vi "CSMOMgr-Get CSMO.vi"(6 "GenError? (T)":bool=TRUE, 8 "Error In":errorcluster caption="error in (no error)", 10 "Queue Name":string, 11 "CSMOMgr":T6) -> (0 "error out":errorcluster, 1 "Values":T1={"info"={"Module Name"="", "Requested Name"="", "Group Name"="", "Mode"=enum."Stand Alone", "Allowed Messages"=[]}, "Refs"={"WatchDogQ"=refnum, "CSMDataDVR"=refnum, "Queue"={"HPriorityQ"=refnum, "LowPriorityQ"=refnum}, "GroupDataDVR"=refnum, "TagMap"=refnum, "ExitEvent"=refnum, "NewStateEvent"=refnum, "StatusEvent"=refnum, "InterruptEvent"=refnum}}, 2 "Found":bool, 3 "CSMOMgr Out":T6)   [LabVIEW 2017, in "Communicable State Machine.lvlib"]
uses:
  Communicable State Machine.lvlib
  Def-CSMOMgr.ctl
  CSMQ/_CSMObj.ctl
  CSMQ/_CSMObj-Info.ctl
  Typedef/_CSM_MODE.ctl
  CSMQ/_CSMObj-Refs.ctl
  CSMQ/_CSMObj-Data.ctl
  Priority Queue/Priority Queue.ctl
  Typedef/_Cross CSM State Data.ctl
  Typedef/_CSM_MSG_TYPE.ctl
  Typedef/_Cross CSM State Response.ctl
  Typedef/_CSM_Response Source Message.ctl
  Priority Queue/def-Data(LowPRI-Q).ctl
  CSMQ/_CSMObj-ModeData.ctl
  Typedef/_CSM Status Change Event Data.ctl
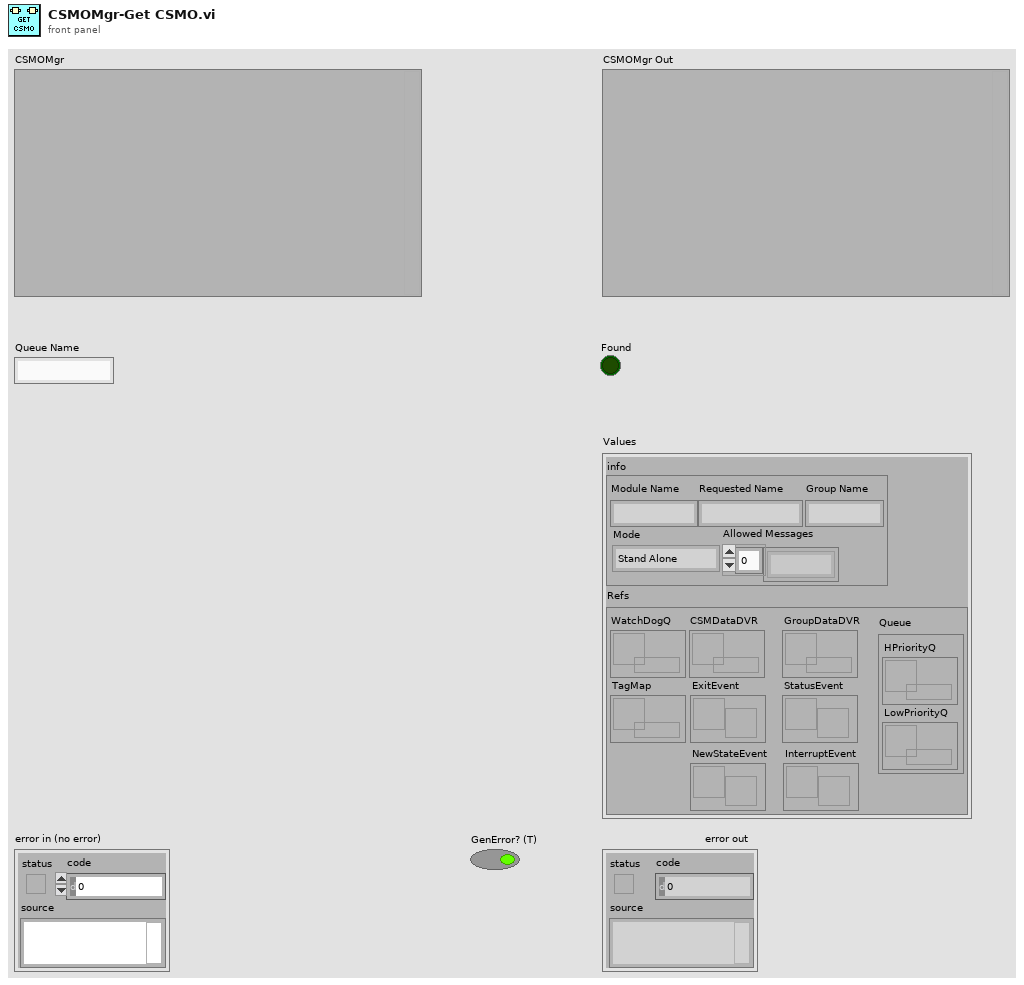
[diagram p1: front panel]
types:
  T1 = typedef "Communicable State Machine.lvlib/_CSMObj.ctl" = cluster{"info":T2, "Refs":T4}
  T2 = typedef "Communicable State Machine.lvlib/_CSMObj-Info.ctl" = cluster{"Module Name":string, "Requested Name":string, "Group Name":string, "Mode":T3, "Allowed Messages":string[]}
  T3 = typedef "Communicable State Machine.lvlib/_CSM_MODE.ctl" = enum16{"Not Exist", "Stand Alone", "CSM", "Worker", "Worker Agent", "Chain Node", "Chain"}
  T4 = typedef "Communicable State Machine.lvlib/_CSMObj-Refs.ctl" = cluster{"WatchDogQ":refnum<queue>, "CSMDataDVR":refnum<data-value>, "Queue":T5, "GroupDataDVR":refnum<data-value>, "TagMap":refnum<data-value>, "ExitEvent":refnum<user-event>, "NewStateEvent":refnum<user-event>, "StatusEvent":refnum<user-event>, "InterruptEvent":refnum<user-event>}
  T5 = typedef "Communicable State Machine.lvlib/Priority Queue.ctl" = cluster{"HPriorityQ":refnum<queue>, "LowPriorityQ":refnum<queue>}
  T6 = typedef "Communicable State Machine.lvlib/Def-CSMOMgr.ctl" = variant
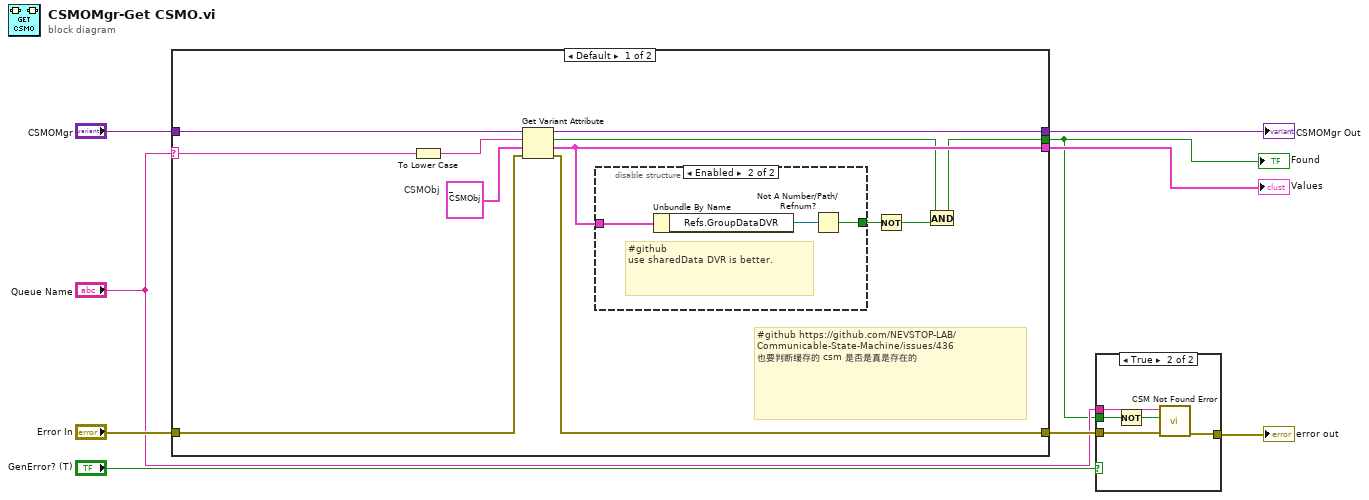
[diagram p0: block diagram]
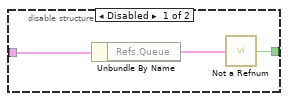
[diagram p3: hidden frame]
diagram:
  n1 = case shown="Default" "Queue Name" {
    selector: "Queue Name" -> [w16 _]
    tunnel: "CSMOMgr" -> [w21 w29]
    tunnel: [w20 w29] -> w8
    tunnel: "Error In" -> [w19 w28]
    tunnel: [w17 w28] -> w6
    tunnel: [w14 _] -> w4
    tunnel: [w13 _] -> w2
    frame Default {
      w18 = T1 {"info"={"Module Name"="", "Requested Name"="", "Group Name"="", "Mode"=enum."Not Exist", "Allowed Messages"=[]}, "Refs"={"WatchDogQ"=refnum, "CSMDataDVR"=refnum, "Queue"={"HPriorityQ"=refnum, "LowPriorityQ"=refnum}, "GroupDataDVR"=refnum, "TagMap"=refnum, "ExitEvent"=refnum, "NewStateEvent"=refnum, "StatusEvent"=refnum, "InterruptEvent"=refnum}}  # CSMObj
      # "#github https://github.com/NEVSTOP-LAB/Communicable-State-Machine/issues/436\n也要判断缓存的 csm 是否是真是存在的"
      n2 = To Lower Case(string=w16) -> (all lower case string=w15:string)
      n3 = Get Variant Attribute(Variant=w21, name=w15, default value (empty Variant)=w18, error in=w19) -> (duplicate Variant=w20:variant, found=w12:bool, value=w14:T1, error out=w17:errorcluster)
      n4 = disable-structure shown="Enabled" {
        disable-tunnel: w14 -> [w24 w27]
        disable-tunnel: [w22 w25] -> w11
        frame Disabled {
          n5 = Unbundle By Name(w24) -> ("Refs.Queue"=w23:T5)
          n6 = call "Not a Refnum.vi"("Priority Queue.lvclass"=w23) -> ("NaN/Path/Refnum?"=w22:bool)  [unwired: 4 in]
        }
        frame Enabled {
          # "#github \nuse sharedData DVR is better."
          n7 = Unbundle By Name(w27) -> ("Refs.GroupDataDVR"=w26:refnum<data-value>)
          n8 = Not A Number/Path/Refnum?(number/path/refnum=w26) -> (NaN/Path/Refnum?=w25:bool)
        }
      }
      n9 = Not(x=w11) -> (.not. x?=w10:bool)
      n10 = And(x=w12, y=w10) -> (x .and. y?=w13:bool)
    }
    frame "" {
    }
  }
  "CSMOMgr Out" <- w8
  "Values" <- w4
  "Found" <- w2
  n11 = case shown="True" "GenError? (T)" {
    tunnel: w6 -> [w30 w35]
    tunnel: [w30 w34] -> w5
    tunnel: "Queue Name" -> [_ w33]
    tunnel: w2 -> [_ w32]
    frame False {
    }
    frame True {
      n12 = Not(x=w32) -> (.not. x?=w31:bool)
      n13 = call "CSM Not Found Error.vi"("error in (no error)"=w35, "Occured?"=w31, "Queue Name"=w33) -> ("error out"=w34:errorcluster)  [unwired: 8 in]
    }
  }
  "error out" <- w5
